vi "FInd Element With Tag.vi"(10 "Tag":string, 11 "Plots":T1[](array[typedef])) -> (2 "Index":i32, 3 "Plot":T1)   [LabVIEW 2017]
uses:
  Typedefs/Plot Data--Cluster.ctl
  Measurement.PhotocurrentMapping.UI.lvclass
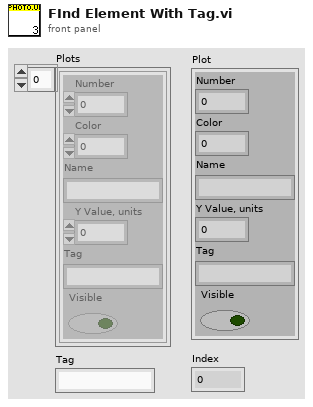
[diagram p1: front panel]
types:
  T1 = typedef "Measurement.PhotocurrentMapping.UI.lvclass/Plot Data--Cluster.ctl" = cluster{"Number":u32, "Color":u32, "Name":string, "Y Value, units":dbl, "Tag":string, "Visible":bool}
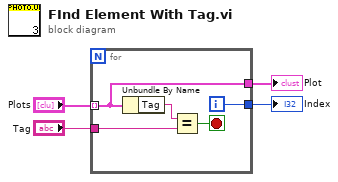
[diagram p0: block diagram]
diagram:
  n1 = for {
    tunnel: "Plots" -> [w7] mode=indexing
    tunnel: "Tag" -> [w8]
    tunnel: [w7] -> w2
    tunnel: [w5] -> w1
    i -> [w5]
    stop <- w6 stop-if-true
    n2 = Unbundle By Name(w7) -> ("Tag"=w9:string)
    n3 = Equal?(x=w9, y=w8) -> (x = y?=w6:bool)
  }
  "Plot" <- w2
  "Index" <- w1
